vi "Query Results Display.vi"(8 "error IO":errorcluster, 11 "VISA resource name":refnum<visa-resource-name>) -> (0 "error Out":errorcluster, 2 "Results Display":enum16{"Last", "ALL", "P/F"}(ring), 3 "VISA resource Out":refnum<visa-resource-name>)   [LabVIEW 2020, in "eec EST 300.lvlib"]
doc: "SR?\nReturns the Results Display setting. There are 3 options:\n\n0=Last: a Results summary screen will be displayed at the end of the test or sequence of connected steps displaying the results of all of the steps.\n1=AllL: the results of the last step performed will be displayed on the Perform Tests screen.\n2=P/F: a Pass or Fail screen will be displayed at the end of the test."
uses:
  <instrlib>/eec EST 300/eec EST 300.lvlib
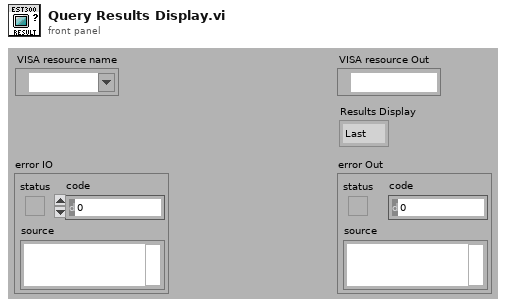
[diagram p1: front panel]
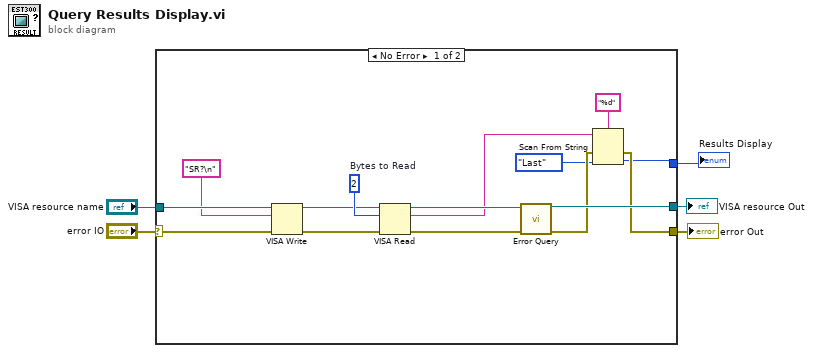
[diagram p0: block diagram]
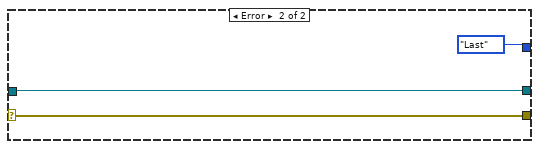
[diagram p2: hidden frame]
diagram:
  n1 = case shown="No Error" "error IO" {
    selector: "error IO" -> [w20 w23]
    tunnel: [w9 w23] -> w2
    tunnel: [w18 w22] -> w3
    tunnel: "VISA resource name" -> [w19 w22]
    tunnel: [w7 enum16{"Last", "ALL", "P/F"}."Last" ("Results Display")] -> w1
    frame No Error {
      w14 = u32 2  # Bytes to Read
      n2 = VISA Write(VISA resource name=w19, write buffer="SR?\n" ("Command to Send (empty)"), error in (no error)=w20) -> (VISA resource name out=w13:refnum<visa-resource-name>, error out=w12:errorcluster)  [unwired: 1 out]
      n3 = VISA Read(VISA resource name=w13, byte count=w14, error in (no error)=w12) -> (VISA resource name out=w16:refnum<visa-resource-name>, read buffer=w8:string, error out=w15:errorcluster)  [unwired: 1 out]
      n4 = call <instrlib>:"Error Query.vi"("VISA resource name"=w16, "error in (no error)"=w15) -> ("VISA resource name out"=w18:refnum<visa-resource-name>, "error out"=w10:errorcluster)  [unwired: 10 in, 2 out]
      n5 = Scan From String(format string="%d", input string=w8, error in=w10, default 1=enum16{"Last", "ALL", "P/F"}."Last" ("Results Display")) -> (error out=w9:errorcluster, output 1=w7:enum16{"Last", "ALL", "P/F"})  [unwired: 1 in, 2 out]
    }
    frame Error {
    }
  }
  "VISA resource Out" <- w3
  "error Out" <- w2
  "Results Display" <- w1
